vi "Calculate Eye Latency.vi"(5 "Onset Indicies":i32[](array[numeric]), 7 "Peak Indicies":i32[](array[numeric]), 8 "error in (no error)":errorcluster, 9 "Response in":dbl[][](array[numeric]), 10 "Stimulus in":dbl[][](array[numeric]), 11 "Head Impulse Fit in":refnum<class "Head Impulse Fit.lvclass">) -> (0 "error out":errorcluster, 1 "Response out":dbl[][](array[numeric]), 2 "Stimulus out":dbl[][](array[numeric]), 3 "Head Impulse Fit out":refnum<class "Head Impulse Fit.lvclass">)   [LabVIEW 2016, in "Head Impulse Fit.lvclass"]
uses:
  Head Impulse Fit.lvclass
  Head Impulse Fit.lvclass/Head Impulse Fit.ctl
  <vilib>/Analysis/1siggen.llb/Ramp Pattern by Delta.vi
  comm/stats/stats.lvlib
  <vilib>/Analysis/NI_AALBase.lvlib
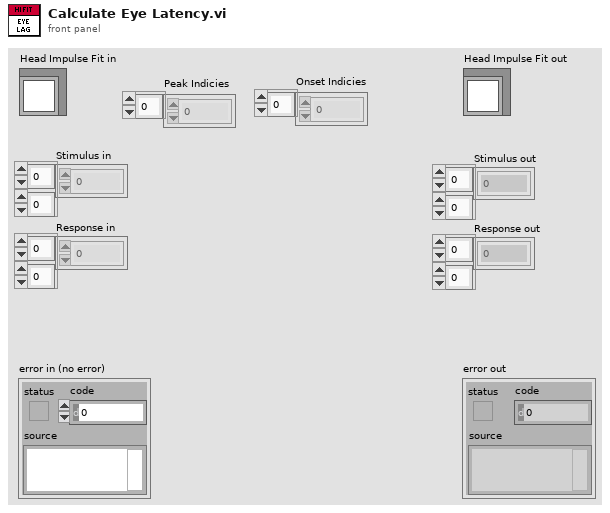
[diagram p1: front panel]
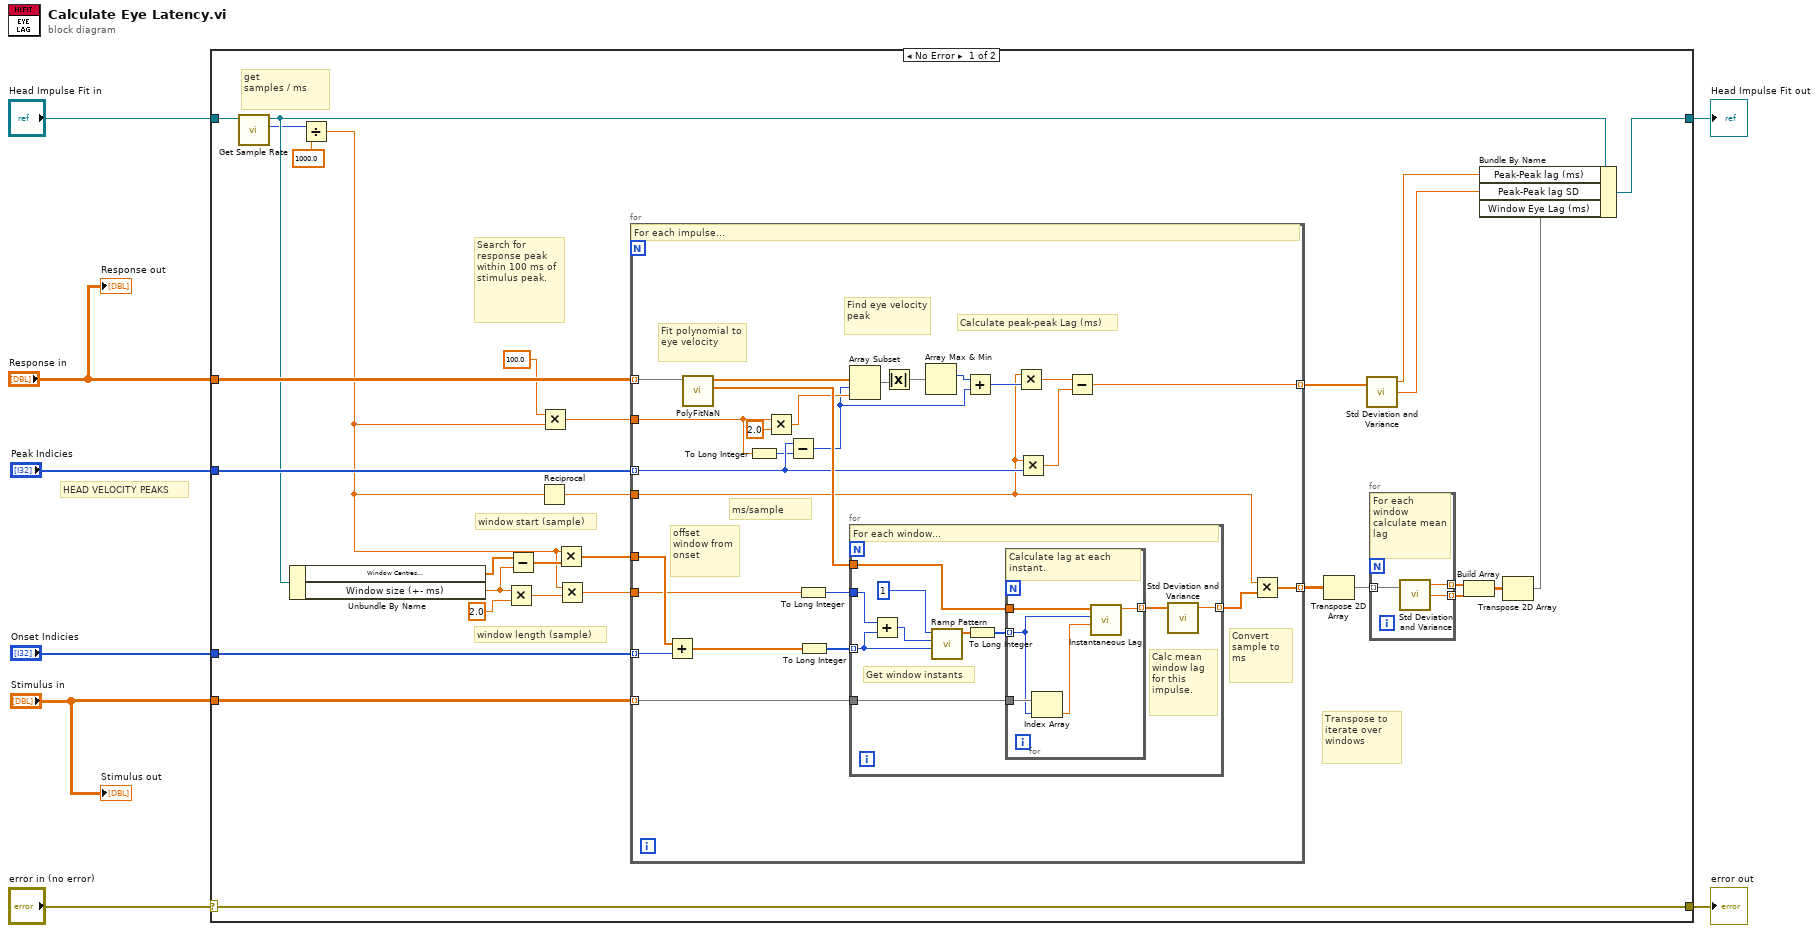
[diagram p0: block diagram]
diagram:
  # "HEAD VELOCITY PEAKS"
  n1 = case shown="No Error" "error in (no error)" {
    selector: "error in (no error)" -> [w38 w84]
    tunnel: [w38 w84] -> w7
    tunnel: [w36 w83] -> w5
    tunnel: "Head Impulse Fit in" -> [w34 w83]
    tunnel: "Peak Indicies" -> [w37 _]
    tunnel: "Response in" -> [w35 _]
    tunnel: "Onset Indicies" -> [w29 _]
    tunnel: "Stimulus in" -> [w22 _]
    frame No Error {
      # "window length (sample)"
      # "window start (sample)"
      # "get\nsamples / ms"
      # "Search for response peak within 100 ms of stimulus peak."
      # "Transpose to iterate over windows"
      n2 = call-dynamic "Get Sample Rate.vi"("Abstract Fit in"=w34) -> ("Sample Rate"=w19:i32, "Abstract Fit out"=w30:refnum<class "Head Impulse Fit.lvclass">)  [unwired: 8 in, 1 out]
      n3 = Unbundle By Name(w30) -> ("Window Centres\n(ms after onset)"=w15:dbl[], "Window size (+- ms)"=w14:dbl)
      n4 = Divide(x=w19, y=1000.0 ("x")) -> (x/y=w11:dbl)
      n5 = Multiply(x=w14, y=2.0) -> (x*y=w12:dbl)
      n6 = Subtract(x=w15, y=w14) -> (x-y=w13:dbl[])
      n7 = Reciprocal(x=w11) -> (1/x=w20:dbl)
      n8 = Multiply(x=100.0 ("y"), y=w11) -> (x*y=w21:dbl)
      n9 = Multiply(x=w11, y=w13) -> (x*y=w10:dbl[])
      n10 = Multiply(x=w11, y=w12) -> (x*y=w9:dbl)
      n11 = for {
        tunnel: w37 -> [w60] mode=indexing
        tunnel: w35 -> [w44] mode=indexing
        tunnel: [w65] -> w33 mode=indexing
        tunnel: w29 -> [w64] mode=indexing
        tunnel: w22 -> [w43] mode=indexing
        tunnel: [w51] -> w28 mode=indexing
        tunnel: w21 -> [w53]
        tunnel: w20 -> [w50]
        tunnel: w9 -> [w46]
        tunnel: w10 -> [w49]
        # "offset window from onset"
        # "ms/sample"
        # "Convert sample to ms"
        # "Calculate peak-peak Lag (ms)"
        # "Find eye velocity peak"
        # "Fit polynomial to eye velocity"
        # "For each impulse..."
        n12 = Add(x=w49, y=w64) -> (x+y=w48:dbl[])
        n13 = call "PolyFitNaN.vi"("Data"=w44) -> ("Polynomial Coefficients"=w62:dbl[], "Best Polynomial Fit"=w42:dbl[])  [unwired: 9 in]
        n14 = To Long Integer(number=w53) -> (32bit integer=w54:i32)
        n15 = Multiply(x=w53, y=2.0) -> (x*y=w58:dbl)
        n16 = Subtract(x=w60, y=w54) -> (x-y=w56:i32)
        n17 = To Long Integer(number=w46) -> (32bit integer=w45:i32)
        n18 = To Long Integer(number=w48) -> (32bit integer=w47:i32[])
        n19 = Array Subset(array=w42, index=w56, length=w58) -> (w63:dbl[])
        n20 = for {
          tunnel: w47 -> [w76] mode=indexing
          tunnel: w43 -> [w74]
          tunnel: w62 -> [w73]
          tunnel: [w71] -> w52 mode=indexing
          tunnel: w45 -> [w77]
          # "Calc mean window lag for this impulse."
          # "Get window instants"
          # "For each window..."
          n21 = Add(x=w77, y=w76) -> (x+y=w75:i32)
          n22 = call-poly <vilib>:"Ramp Pattern.vi"("start"=w76, "end"=w75, "delta"=1) -> ("Ramp Pattern"=w70:dbl[])  [unwired: 6 in, 2 out]
          n23 = To Long Integer(number=w70) -> (32bit integer=w68:i32[])
          n24 = for {
            tunnel: w68 -> [w80] mode=indexing
            tunnel: w74 -> [w81]
            tunnel: w73 -> [w82]
            tunnel: [w78] -> w72 mode=indexing
            # "Calculate lag at each instant."
            n25 = Index Array(array=w81, index=w80) -> (element=w79:dbl)
            n26 = call "Instantaneous Lag.vi"("Instant Stimulus Value"=w79, "Instant (sample)"=w80, "Response Polynomial Coefficients"=w82) -> ("Instant Response Lag (sample)"=w78:dbl)  [unwired: 7 in, 1 out]
          }
          n27 = call "Std Deviation and Variance.vi"("X"=w72) -> ("mean"=w71:dbl)  [unwired: 1 in, 2 out]
        }
        n28 = Absolute Value(x=w63) -> (abs(x)=w61:dbl[])
        n29 = Array Max & Min(array=w61) -> (max index (indices)=w57:i32)  [unwired: 3 out]
        n30 = Add(x=w57, y=w56) -> (x+y=w55:i32)
        n31 = Multiply(x=w50, y=w55) -> (x*y=w67:dbl)
        n32 = Multiply(x=w50, y=w60) -> (x*y=w66:dbl)
        n33 = Subtract(x=w67, y=w66) -> (x-y=w65:dbl)
        n34 = Multiply(x=w50, y=w52) -> (x*y=w51:dbl[])
      }
      n35 = Transpose 2D Array(2D array=w28) -> (transposed array=w27:dbl[][])
      n36 = call "Std Deviation and Variance.vi"("X"=w33) -> ("mean"=w32:dbl, "standard deviation"=w31:dbl)  [unwired: 1 in, 1 out]
      n37 = for {
        tunnel: w27 -> [w41] mode=indexing
        tunnel: [w40] -> w26 mode=indexing
        tunnel: [w39] -> w25 mode=indexing
        # "For each window calculate mean lag"
        n38 = call "Std Deviation and Variance.vi"("X"=w41) -> ("mean"=w40:dbl, "standard deviation"=w39:dbl)  [unwired: 1 in, 1 out]
      }
      n39 = Build Array(w26, w25) -> (w24:dbl[][])
      n40 = Transpose 2D Array(2D array=w24) -> (transposed array=w23:dbl[][])
      n41 = Bundle By Name(cluster=w30, "Peak-Peak lag (ms)"=w32, "Peak-Peak lag SD"=w31, "Window Eye Lag (ms)"=w23) -> (w36:refnum<class "Head Impulse Fit.lvclass">)
    }
    frame Error {
    }
  }
  "error out" <- w7
  "Head Impulse Fit out" <- w5
  "Response out" <- "Response in"
  "Stimulus out" <- "Stimulus in"
